vi "String.vi"() -> ()   [LabVIEW 2023]
uses:
  <vilib>/regexp/Match Regular Expression.xnode
panel:
  out "이후 부분 문자열":string
  out "길이":i32
  in  "맺음말":string
  in  "머릿말":string
  out "결과문":string
  out "점수":string
  out "결과":dbl
  in  "난이도":dbl
  in  "독창성":dbl
  in  "창의력":dbl
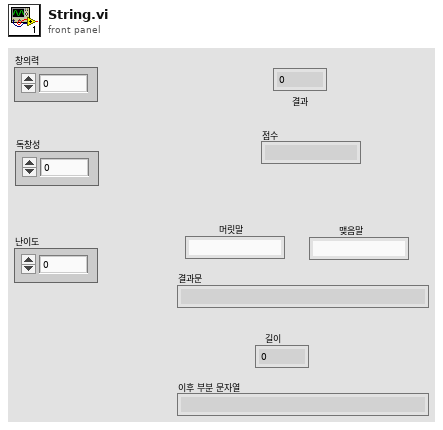
[diagram p1: front panel]
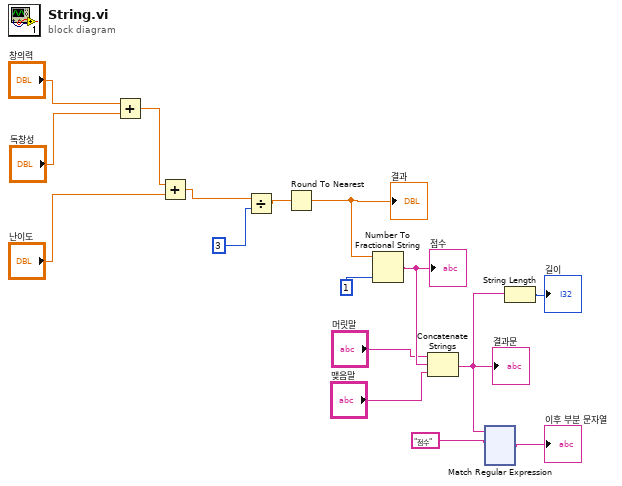
[diagram p0: block diagram]
diagram:
  n1 = Add(x="창의력", y="독창성") -> (x+y=w13:dbl)
  n2 = Add(x=w13, y="난이도") -> (x+y=w12:dbl)
  n3 = Divide(x=w12, y=3) -> (x/y=w10:dbl)
  n4 = Round To Nearest(number=w10) -> (nearest integer value=w9:dbl)
  "결과" <- w9
  n5 = Number To Fractional String(number=w9, precision (6)=i16 1) -> (F-format string=w7:string)  [unwired: 2 in]
  "점수" <- w7
  n6 = Concatenate Strings("머릿말", w7, "맺음말") -> (w1:string)
  "결과문" <- w1
  n7 = xnode "Match Regular Expression"("input string"=w1, "regular expression"="점수") -> ("after match"=→"이후 부분 문자열":string)  [unwired: 4 in, 4 out]
  n8 = String Length(string=w1) -> (length=→"길이":i32)
